vi "PH_TKTDS-30xx.Evt Call Fetch Waveform.vi"(0 "i ref in":refnum<vi>, 1 "Instance":string="N/A", 2 "Waveform to fetch":T1={"Source"="CH1", "Waveform Start"=10000, "Waveform End"=0}, 5 "error in (no error)":errorcluster) -> (14 "i ref out":refnum<vi>, 19 "error out":errorcluster)   [LabVIEW 2014, in "PH_TKTDS-30xx.lvlib"]
doc: "This VI calls sets a simple call."
uses:
  PH_TKTDS-30xx.lvlib
  PH_TKTDS-30xx.Waveform to fetch.ctl
  CS_Core/CSSystem/CoreLib/CoreLib.int 2 byte array.vi
  CS_Core/CSSystem/CoreLib/CoreLib.string 2 byte array.vi
  CS_Core/CSSystem/CoreLib/CoreLib.lvlib
  CS_Core/BaseProcess/BaseProcess.lvlib
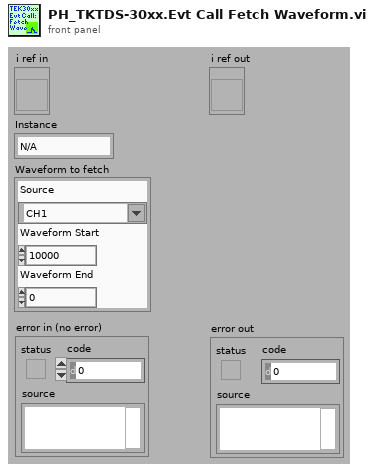
[diagram p1: front panel]
types:
  T1 = typedef "PH_TKTDS-30xx.lvlib/PH_TKTDS-30xx.Waveform to fetch.ctl" = cluster{"Source":string, "Waveform Start":i32, "Waveform End":i32}
  T2 = typedef "CoreDefs.rawDataType.ctl" = i8[]
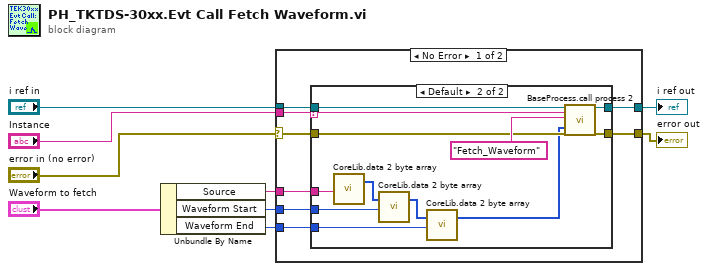
[diagram p0: block diagram]
diagram:
  n1 = Unbundle By Name("Waveform to fetch") -> ("Source"=w3:string, "Waveform Start"=w2:i32, "Waveform End"=w1:i32)
  n2 = case shown="No Error" "error in (no error)" {
    selector: "error in (no error)" -> [w13 w32]
    tunnel: [w17 w33] -> w9
    tunnel: [w16 w32] -> w8
    tunnel: "i ref in" -> [w15 w33]
    tunnel: w3 -> [w12 _]
    tunnel: "Instance" -> [w14 _]
    tunnel: w2 -> [w11 _]
    tunnel: w1 -> [w10 _]
    frame No Error {
      n3 = case shown="Default" w14 {
        selector: w14 -> [_ w26]
        tunnel: [w18 w30] -> w17
        tunnel: [w19 w29] -> w16
        tunnel: w15 -> [w18 w28]
        tunnel: w13 -> [w19 w27]
        tunnel: w12 -> [_ w25]
        tunnel: w11 -> [_ w21]
        tunnel: w10 -> [_ w23]
        frame "N/A" {
        }
        frame Default {
          n4 = call-poly "CoreLib.data 2 byte array.vi"("string"=w25) -> ("byteArray out"=w24:T2)  [unwired: 18 in]
          n5 = call-poly "CoreLib.data 2 byte array.vi"("byteArray"=w24, "i32"=w21) -> ("byteArray out"=w22:T2)  [unwired: 17 in]
          n6 = call-poly "CoreLib.data 2 byte array.vi"("byteArray"=w22, "i32"=w23) -> ("byteArray out"=w20:T2)  [unwired: 17 in]
          n7 = call "BaseProcess.call process 2.vi"("i ref in"=w28, "Object"=w26, "Selector"="Fetch_Waveform", "Data"=w20, "error in (no error)"=w27) -> ("i ref out"=w30:refnum<vi>, "error out"=w29:errorcluster)  [unwired: 13 in]
        }
      }
    }
    frame Error {
    }
  }
  "i ref out" <- w9
  "error out" <- w8
